vi "18-Reduce.vi"(11 "Snailfish Number in":string) -> (3 "Snailfish Number out":string)   [LabVIEW 2019, in "18.lvlib"]
uses:
  18.lvlib
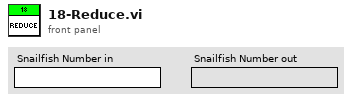
[diagram p1: front panel]
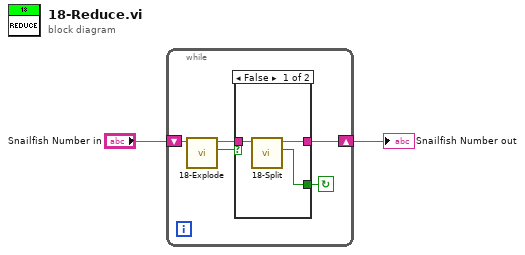
[diagram p0: block diagram]
diagram:
  n1 = while {
    shift-right: [w5] -> w2
    shift-left: "Snailfish Number in" -> [w7]
    stop <- w4 continue-if-true
    n2 = call "18-Explode.vi"("Snailfish Number in"=w7) -> ("Exploded?"=w3:bool, "Snailfish Number out"=w6:string)  [unwired: 9 in]
    n3 = case shown="False" w3 {
      selector: w3 -> [_ w12]
      tunnel: w6 -> [w8 w11]
      tunnel: [w9 w11] -> w5
      tunnel: [w10 w12] -> w4
      frame False {
        n4 = call "18-Split.vi"("Snailfish Number in"=w8) -> ("Split?"=w10:bool, "Snailfish Number out"=w9:string)  [unwired: 9 in]
      }
      frame True {
      }
    }
  }
  "Snailfish Number out" <- w2
